vi "Begin.vi"(8 "error in":errorcluster) -> (0 "error out":errorcluster)   [LabVIEW 2017]
doc: "Called before other user functions, this VI is expected to open initial I/O refnums, load in file data, and do all program initialization. Notice that the <B>error out</B> terminal is simply used for data flow. Wiring it to other structures or subVIs ensures that this VI runs first."
uses:
  <vilib>/Rock Robotics/SystemInterfaces/DIO/FPGA_DIOPWMChannel.ctl
  <vilib>/Rock Robotics/WPI/SafetyOutput/WPI_SafetyOutputConfigMenu.ctl
  <vilib>/Rock Robotics/WPI/DriverStation/WPI_DriverStationRobotMode2.ctl
  <vilib>/Rock Robotics/WPI/Joystick/WPI_JoystickDeviceEnum.ctl
  <vilib>/Rock Robotics/WPI/Solenoid/WPI_SolenoidChannel.ctl
  <vilib>/Rock Robotics/SystemInterfaces/DIO/FPGA_DIOChannel.ctl
  <vilib>/Rock Robotics/WPI/Encoder/WPI_EncoderType.ctl
  Robot Global Data.vi
  <vilib>/Rock Robotics/Network Tables/NT Write String Array.vi
  <vilib>/Rock Robotics/WPI/RobotDrive/WPI_RobotDriveOpen4MotorWithSPARK.vi
  <vilib>/Rock Robotics/WPI/MotorControl/WPI_MotorControlOpen SPARK.vi
  <vilib>/Rock Robotics/WPI/Solenoid/WPI_SolenoidOpenSingle.vi
  <vilib>/Rock Robotics/WPI/Utilities/WPI_GetSetVariantRefNum.vi
  <vilib>/Rock Robotics/WPI/Counter/WPI_CounterDigitalInputToDigitalSource.vi
panel:
  out "Comp. Running":bool
  out "Enabled":bool
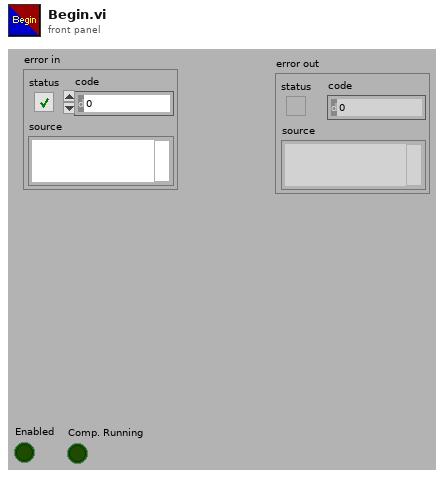
[diagram p1: front panel]
types:
  T1 = typedef "FPGA_DIOChannel.ctl" = enum8{"DIO 0", "DIO 1", "DIO 2", "DIO 3", "DIO 4", "DIO 5", "DIO 6", "DIO 7", "DIO 8", "DIO 9", "DIO MXP 0", "DIO MXP 1", "DIO MXP 2", "DIO MXP 3", "DIO MXP 4", "DIO MXP 5", "DIO MXP 6", "DIO MXP 7", "DIO MXP 8", "DIO MXP 9", "DIO MXP 10", "DIO MXP 11", "DIO MXP 12", "DIO MXP 13", "DIO MXP 14", "DIO MXP 15", "SPI Port CS1", "SPI Port CS2", "SPI Port CS3", "SPI Port MISO", "SPI Port MOSI", "Invalid"}
  T2 = typedef "WPI_EncoderType.ctl" = enum16{"1x", "2x", "4x"}
  T3 = typedef "WPI_SolenoidChannel.ctl" = enum8{"Solenoid 0", "Solenoid 1", "Solenoid 2", "Solenoid 3", "Solenoid 4", "Solenoid 5", "Solenoid 6", "Solenoid 7", "Invalid"}
  T4 = typedef "FPGA_DIOPWMChannel.ctl" = enum8{"PWM 0", "PWM 1", "PWM 2", "PWM 3", "PWM 4", "PWM 5", "PWM 6", "PWM 7", "PWM 8", "PWM 9", "PWM MXP 0", "PWM MXP 1", "PWM MXP 2", "PWM MXP 3", "PWM MXP 4", "PWM MXP 5", "PWM MXP 6", "PWM MXP 7", "PWM MXP 8", "PWM MXP 9", "Invalid"}
  T5 = typedef "WPI_JoystickDeviceEnum.ctl" = enum16{"USB 0", "USB 1", "USB 2", "USB 3", "USB 4", "USB 5"}
  T6 = typedef "WPI_DriverStationRobotMode2.ctl" = enum16{"Autonomous Disabled", "Autonomous Enabled", "Teleop Disabled", "Teleop Enabled", "Disconnected", "Finish", "Test Disabled", "Test Enabled", "Emergency Stopped"}
  T7 = typedef "WPI_SafetyOutputConfigMenu.ctl" = enum16{"Enable", "Disable"}
  T8 = typedef "WPI_DigitalInputDevRef.ctl" = cluster{"DevStatus":errorcluster, "DIO Channel":T1}
  T9 = typedef "FPGA_CounterEncoderSourceConvertionLVSourceType.ctl" = cluster{"DevStatus":errorcluster, "AnalogTriggerMode?":bool, "DigitalMode":cluster{"DIO Channel":T10}, "AnalogTriggerMode":cluster{"AnalogTriggerIndex":T11, "OutputType":T12}}
  T10 = typedef "FPGA_DIODigitalSourceChannel.ctl" = enum8{"DIO 0", "DIO 1", "DIO 2", "DIO 3", "DIO 4", "DIO 5", "DIO 6", "DIO 7", "DIO 8", "DIO 9", "DIO MXP 0", "DIO MXP 1", "DIO MXP 2", "DIO MXP 3", "DIO MXP 4", "DIO MXP 5", "DIO MXP 6", "DIO MXP 7", "DIO MXP 8", "DIO MXP 9", "DIO MXP 10", "DIO MXP 11", "DIO MXP 12", "DIO MXP 13", "DIO MXP 14", "DIO MXP 15", "Disabled"}
  T11 = typedef "FPGA_AnalogTriggerIndex.ctl" = enum8{"Trig 0", "Trig 1", "Trig 2", "Trig 3", "Trig 4", "Trig 5", "Trig 6", "Trig 7", "Invalid"}
  T12 = typedef "FPGA_AnalogTriggerOutType.ctl" = enum16{"InWindow", "TriggerState", "Rising", "Falling"}
  T13 = typedef "WPI_MotorControlDeviceRef.ctl" = cluster{"DeviceStatus":errorcluster, "Type":T14, "PWM":cluster{"PWM Channel":T4, "DeadBand":T15}, "CAN":cluster{"Device Number":u8, "SetOutput VI Ref":variant, "GetOutput VI Ref":variant, "Enable VI Ref":variant, "Disable VI Ref":variant, "Data":variant}, "Invert":bool, "DIO PWM":cluster{"PWM \"Enable\" Channel":T4, "DIOChannel":T1, "PWM Rate":dbl}}
  T14 = typedef "WPI_MotorControlType.ctl" = enum16{"PWM", "CAN", "DIO PWM"}
  T15 = typedef "WPI_PWMDeadband.ctl" = cluster{"Name":string, "maxPositivePwm":i32, "minPositivePwm":i32, "centerPwm":i32, "maxNegativePwm":i32, "minNegativePwm":i32, "angularRange":u16}
  T16 = typedef "WPI_EncoderDevRef.ctl" = cluster{"DevStatus":errorcluster, "EncoderIndex":T17, "CounterIndex":T18, "DistancePerCount":dbl, "Decoding Type":T2}
  T17 = typedef "FPGA_EncoderIdx.ctl" = enum8{"Enc 0", "Enc 1", "Enc 2", "Enc 3", "Enc 4", "Enc 5", "Enc 6", "Enc 7", "Invalid"}
  T18 = typedef "FPGA_CounterCtrSystemIndex.ctl" = enum8{"Ctr 0", "Ctr 1", "Ctr 2", "Ctr 3", "Ctr 4", "Ctr 5", "Ctr 6", "Ctr 7", "Invalid"}
  T19 = typedef "WPI_RobotDriveDevRef.ctl" = cluster{"DevStatus":errorcluster, "Motors[]":T13[], "Square Inputs":bool, "Max Output":dbl}
  T20 = typedef "WPI_CompressorDevRef.ctl" = cluster{"DevStatus":errorcluster, "Pneumatics Control Module":u8}
  T21 = typedef "WPI_SolenoidDevRef.ctl" = cluster{"DevStatus":errorcluster, "Pneumatics Control Module":u8, "Forward Solenoid Channel":T3, "Reverse Solenoid Channel":T3}
  T22 = typedef "WPI_JoystickDevRef.ctl" = cluster{"Device":T5}
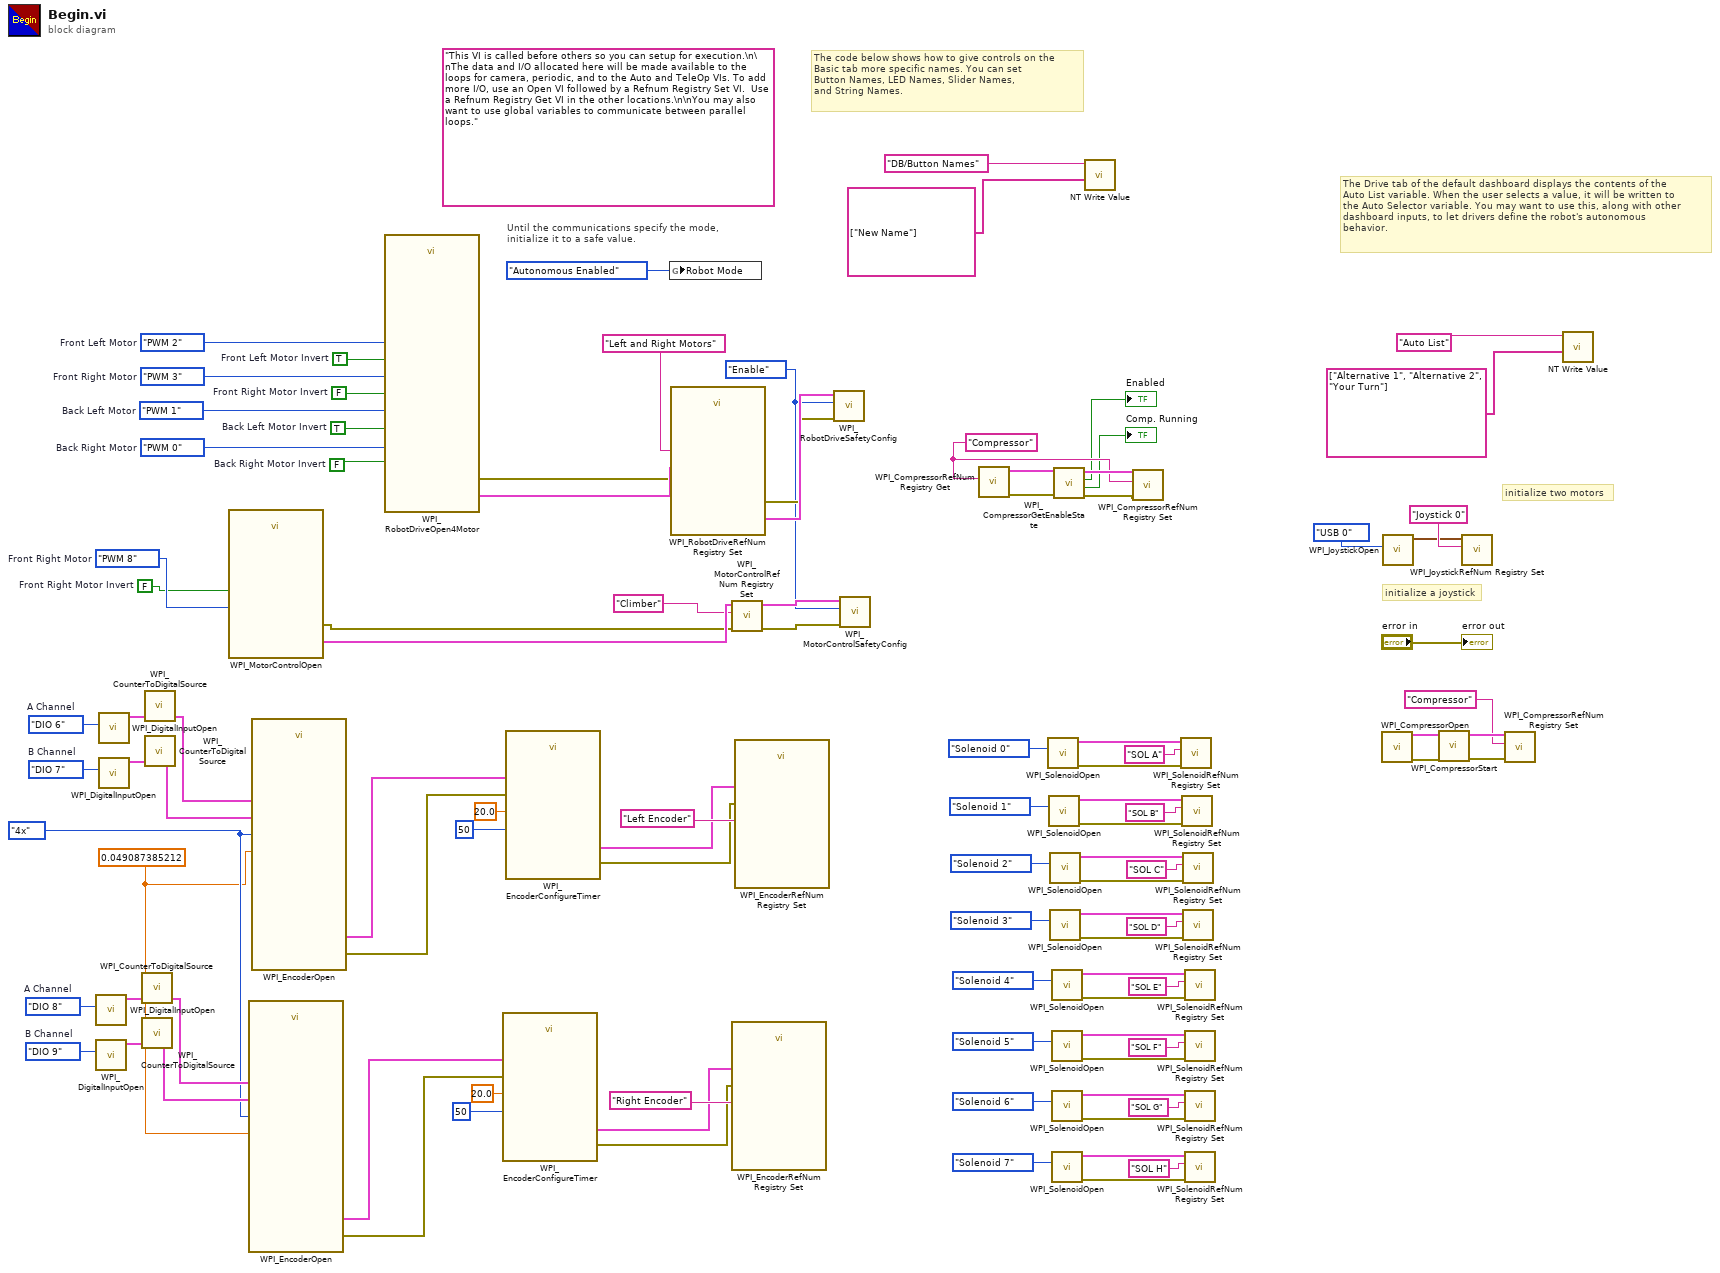
[diagram p0: block diagram]
diagram:
  w1 = 0.049087385212
  w15 = FPGA_DIOChannel."DIO 9"  # B Channel
  w14 = FPGA_DIOChannel."DIO 8"  # A Channel
  w2 = WPI_EncoderType."4x" ("Decoding Type")
  w28 = FPGA_DIOChannel."DIO 7"  # B Channel
  w27 = FPGA_DIOChannel."DIO 6"  # A Channel
  w31 = "Compressor"
  w80 = FALSE  # Front Right Motor Invert
  w81 = FPGA_DIOPWMChannel."PWM 8"  # Front Right Motor
  w36 = FALSE  # Front Right Motor Invert
  w37 = TRUE  # Front Left Motor Invert
  w38 = TRUE  # Back Left Motor Invert
  w39 = FALSE  # Back Right Motor Invert
  w88 = FPGA_DIOPWMChannel."PWM 3"  # Front Right Motor
  w89 = FPGA_DIOPWMChannel."PWM 2"  # Front Left Motor
  w82 = WPI_SafetyOutputConfigMenu."Enable" ("mode")
  (unwired) "This VI is called before others so you can setup for execution.\n\nThe data and I/O allocated here will be made available to the loops for camera, periodic, and to the Auto and TeleOp VIs. To add more I/O, use an Open VI followed by a Refnum Registry Set VI.  Use a Refnum Registry Get VI in the other locations.\n\nYou may also want to use global variables to communicate between parallel loops."
  w40 = FPGA_DIOPWMChannel."PWM 1"  # Back Left Motor
  w41 = FPGA_DIOPWMChannel."PWM 0"  # Back Right Motor
  # "The Drive tab of the default dashboard displays the contents of the\nAuto List variable. When the user selects a value, it will be written to\nthe Auto Selector variable. You may want to use this, along with other\ndashboard inputs, to let drivers define the robot's autonomous\nbehavior."
  # "The code below shows how to give controls on the\nBasic tab more specific names. You can set\nButton Names, LED Names, Slider Names,\nand String Names."
  # "initialize a joystick"
  # "Until the communications specify the mode,\ninitialize it to a safe value."
  # "initialize two motors"
  n1 = call <vilib>:"WPI_DigitalInputOpen.vi"("DIO Channel"=w14) -> ("DigitalInputDevRef"=w11:T8)  [unwired: 1 in, 9 out]
  n2 = call <vilib>:"WPI_DigitalInputOpen.vi"("DIO Channel"=w15) -> ("DigitalInputDevRef"=w12:T8)  [unwired: 1 in, 9 out]
  n3 = call <vilib>:"WPI_DigitalInputOpen.vi"("DIO Channel"=w27) -> ("DigitalInputDevRef"=w24:T8)  [unwired: 1 in, 9 out]
  n4 = call <vilib>:"WPI_DigitalInputOpen.vi"("DIO Channel"=w28) -> ("DigitalInputDevRef"=w25:T8)  [unwired: 1 in, 9 out]
  n5 = call-poly <vilib>:"WPI_CounterToDigitalSource.vi"("DigitalInputDevRef"=w11) -> ("Digital Source"=w10:T9)  [unwired: 6 out]
  n6 = call-poly <vilib>:"WPI_CounterToDigitalSource.vi"("DigitalInputDevRef"=w12) -> ("Digital Source"=w13:T9)  [unwired: 6 out]
  n7 = call-poly <vilib>:"WPI_CounterToDigitalSource.vi"("DigitalInputDevRef"=w24) -> ("Digital Source"=w23:T9)  [unwired: 6 out]
  n8 = call-poly <vilib>:"WPI_CounterToDigitalSource.vi"("DigitalInputDevRef"=w25) -> ("Digital Source"=w26:T9)  [unwired: 6 out]
  n9 = call-poly <vilib>:"WPI_MotorControlOpen.vi"("Invert"=w80, "PWM Channel"=w81) -> ("error out"=w84:errorcluster, "MotorControlDeviceRef"=w86:T13)  [unwired: 8 in]
  n10 = call <vilib>:"WPI_EncoderOpen.vi"("DistancePerCount"=w1, "Decoding Type"=w2, "BSource"=w13, "ASource"=w10) -> ("error out"=w4:errorcluster, "EncoderDevRef"=w8:T16)  [unwired: 4 in, 2 out]
  n11 = call <vilib>:"WPI_EncoderOpen.vi"("DistancePerCount"=w1, "Decoding Type"=w2, "BSource"=w26, "ASource"=w23) -> ("error out"=w17:errorcluster, "EncoderDevRef"=w21:T16)  [unwired: 4 in, 2 out]
  n12 = call-poly <vilib>:"WPI_RobotDriveOpen4Motor.vi"("Rear Left Motor"=w40, "Rear Left Motor Inverted"=w38, "Rear Right Motor Inverted"=w39, "Rear Right Motor"=w41, "Front Left Motor"=w89, "Front Right Motor"=w88, "Front Left Motor Inverted"=w37, "Front Right Motor Inverted"=w36) -> ("RobotDriveDevRef"=w91:T19, "error out"=w90:errorcluster)  [unwired: 6 in]
  n13 = call <vilib>:"WPI_EncoderConfigureTimer.vi"("error in (no error)"=w4, "Number Samples to Average"=u8 50, "Minimum Rate"=20.0, "EncoderDevRef"=w8) -> ("error out"=w3:errorcluster, "EncoderDevRef"=w7:T16)  [unwired: 6 in]
  n14 = call <vilib>:"WPI_EncoderConfigureTimer.vi"("error in (no error)"=w17, "Number Samples to Average"=u8 50, "Minimum Rate"=20.0, "EncoderDevRef"=w21) -> ("error out"=w16:errorcluster, "EncoderDevRef"=w20:T16)  [unwired: 6 in]
  n15 = global write "Robot Global Data.vi" "Robot Mode"(WPI_DriverStationRobotMode2."Autonomous Enabled" ("Robot Mode")) -> ()
  n16 = call <vilib>:"WPI_RobotDriveRefNum Registry Set.vi"("error in (no error)"=w90, "refnum name"="Left and Right Motors", "RobotDriveDevRef"=w91) -> ("error out"=w87:errorcluster, "RobotDriveDevRef"=w101:T19)  [unwired: 1 in, 6 out]
  n17 = call <vilib>:"WPI_MotorControlRefNum Registry Set.vi"("error in (no error)"=w84, "refnum name"="Climber", "MotorControlDevRef"=w86) -> ("error out"=w83:errorcluster, "MotorControlDevRef"=w85:T13)  [unwired: 7 in]
  n18 = call <vilib>:"WPI_EncoderRefNum Registry Set.vi"("error in (no error)"=w3, "refnum name"="Right Encoder", "EncoderDevRef"=w7) -> ()  [unwired: 7 in, 2 out]
  n19 = call <vilib>:"WPI_EncoderRefNum Registry Set.vi"("error in (no error)"=w16, "refnum name"="Left Encoder", "EncoderDevRef"=w20) -> ()  [unwired: 7 in, 2 out]
  n20 = call <vilib>:"WPI_RobotDriveSafetyConfig.vi"("error in (no error)"=w87, "mode"=w82, "RobotDriveDevRef"=w101) -> ()  [unwired: 7 in, 2 out]
  n21 = call <vilib>:"WPI_MotorControlSafetyConfig.vi"("error in (no error)"=w83, "mode"=w82, "MotorControlDevRef"=w85) -> ()  [unwired: 7 in, 2 out]
  n22 = call <vilib>:"WPI_CompressorRefNum Registry Get.vi"("refnum name"=w31) -> ("error out"=w33:errorcluster, "CompressorDevRef"=w35:T20)  [unwired: 9 in]
  n23 = call-poly <vilib>:"WPI_SolenoidOpen.vi"("Solenoid Channel"=WPI_SolenoidChannel."Solenoid 0") -> ("error out"=w71:errorcluster, "SolenoidDevRef"=w72:T21)  [unwired: 9 in]
  n24 = call-poly <vilib>:"WPI_SolenoidOpen.vi"("Solenoid Channel"=WPI_SolenoidChannel."Solenoid 1") -> ("error out"=w67:errorcluster, "SolenoidDevRef"=w68:T21)  [unwired: 9 in]
  n25 = call-poly <vilib>:"WPI_SolenoidOpen.vi"("Solenoid Channel"=WPI_SolenoidChannel."Solenoid 2") -> ("error out"=w63:errorcluster, "SolenoidDevRef"=w64:T21)  [unwired: 9 in]
  n26 = call-poly <vilib>:"WPI_SolenoidOpen.vi"("Solenoid Channel"=WPI_SolenoidChannel."Solenoid 3") -> ("error out"=w59:errorcluster, "SolenoidDevRef"=w60:T21)  [unwired: 9 in]
  n27 = call-poly <vilib>:"WPI_SolenoidOpen.vi"("Solenoid Channel"=WPI_SolenoidChannel."Solenoid 4") -> ("error out"=w55:errorcluster, "SolenoidDevRef"=w56:T21)  [unwired: 9 in]
  n28 = call-poly <vilib>:"WPI_SolenoidOpen.vi"("Solenoid Channel"=WPI_SolenoidChannel."Solenoid 5") -> ("error out"=w51:errorcluster, "SolenoidDevRef"=w52:T21)  [unwired: 9 in]
  n29 = call-poly <vilib>:"WPI_SolenoidOpen.vi"("Solenoid Channel"=WPI_SolenoidChannel."Solenoid 6") -> ("error out"=w47:errorcluster, "SolenoidDevRef"=w48:T21)  [unwired: 9 in]
  n30 = call-poly <vilib>:"WPI_SolenoidOpen.vi"("Solenoid Channel"=WPI_SolenoidChannel."Solenoid 7") -> ("error out"=w43:errorcluster, "SolenoidDevRef"=w44:T21)  [unwired: 9 in]
  n31 = call <vilib>:"WPI_CompressorGetEnableState.vi"("error in (no error)"=w33, "CompressorDevRef"=w35) -> ("error out"=w32:errorcluster, "Compressor Running"=→"Comp. Running":bool, "Enabled"=→"Enabled":bool, "CompressorDevRef"=w34:T20)  [unwired: 6 in]
  n32 = call-poly <vilib>:"NT Write Value.vi"("String Array"=string[] ["New Name"], "Name"="DB/Button Names") -> ()  [unwired: 9 in, 1 out]
  n33 = call <vilib>:"WPI_CompressorRefNum Registry Set.vi"("error in (no error)"=w32, "refnum name"=w31, "CompressorDevRef"=w34) -> ()  [unwired: 7 in, 2 out]
  n34 = call <vilib>:"WPI_SolenoidRefNum Registry Set.vi"("error in (no error)"=w71, "refnum name"="SOL A", "SolenoidDevRef"=w72) -> ()  [unwired: 7 in, 2 out]
  n35 = call <vilib>:"WPI_SolenoidRefNum Registry Set.vi"("error in (no error)"=w67, "refnum name"="SOL B", "SolenoidDevRef"=w68) -> ()  [unwired: 7 in, 2 out]
  n36 = call <vilib>:"WPI_SolenoidRefNum Registry Set.vi"("error in (no error)"=w63, "refnum name"="SOL C", "SolenoidDevRef"=w64) -> ()  [unwired: 7 in, 2 out]
  n37 = call <vilib>:"WPI_SolenoidRefNum Registry Set.vi"("error in (no error)"=w59, "refnum name"="SOL D", "SolenoidDevRef"=w60) -> ()  [unwired: 7 in, 2 out]
  n38 = call <vilib>:"WPI_SolenoidRefNum Registry Set.vi"("error in (no error)"=w55, "refnum name"="SOL E", "SolenoidDevRef"=w56) -> ()  [unwired: 7 in, 2 out]
  n39 = call <vilib>:"WPI_SolenoidRefNum Registry Set.vi"("error in (no error)"=w51, "refnum name"="SOL F", "SolenoidDevRef"=w52) -> ()  [unwired: 7 in, 2 out]
  n40 = call <vilib>:"WPI_SolenoidRefNum Registry Set.vi"("error in (no error)"=w47, "refnum name"="SOL G", "SolenoidDevRef"=w48) -> ()  [unwired: 7 in, 2 out]
  n41 = call <vilib>:"WPI_SolenoidRefNum Registry Set.vi"("error in (no error)"=w43, "refnum name"="SOL H", "SolenoidDevRef"=w44) -> ()  [unwired: 7 in, 2 out]
  n42 = call <vilib>:"WPI_CompressorOpen.vi"() -> ("CompressorDevRef"=w77:T20, "error out"=w78:errorcluster)  [unwired: 14 in]
  n43 = call <vilib>:"WPI_JoystickOpen.vi"("JoystickDevice"=WPI_JoystickDeviceEnum."USB 0") -> ("JoystickDevRef"=w98:T22)  [unwired: 10 in]
  n44 = call <vilib>:"WPI_CompressorStart.vi"("error in (no error)"=w78, "CompressorDevRef"=w77) -> ("error out"=w75:errorcluster, "CompressorDevRef"=w76:T20)  [unwired: 8 in]
  n45 = call <vilib>:"WPI_JoystickRefNum Registry Set.vi"("refnum name"="Joystick 0", "JoystickDevRef"=w98) -> ()  [unwired: 8 in, 2 out]
  n46 = call <vilib>:"WPI_CompressorRefNum Registry Set.vi"("error in (no error)"=w75, "refnum name"="Compressor", "CompressorDevRef"=w76) -> ()  [unwired: 7 in, 2 out]
  n47 = call-poly <vilib>:"NT Write Value.vi"("String Array"=string[] ["Alternative 1", "Alternative 2", "Your Turn"], "Name"="Auto List") -> ()  [unwired: 9 in, 1 out]
  "error out" <- "error in"
